vi "CONVERSION.vi"(1 "V1":dbl, 2 "B":dbl, 3 "A":dbl) -> (0 "Temp":dbl)   [LabVIEW 2014]
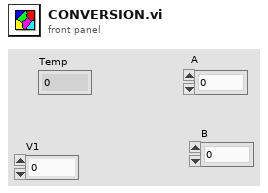
[diagram p1: front panel]
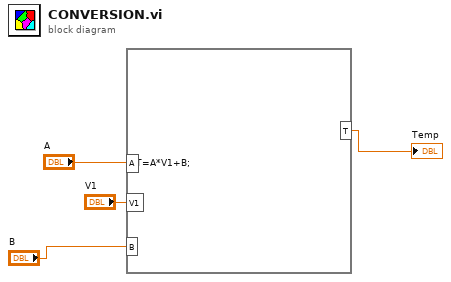
[diagram p0: block diagram]
diagram:
  n1 = formula code="T=A*V1+B;"("A"="A", "V1"="V1", "B"="B") -> ("T"=→"Temp":dbl)
